vi "Markers.vi"(8 "error in (no error)":errorcluster, 10 "Subject Name":string, 11 ".NET Refnum in":refnum<k24>) -> (0 "error out":errorcluster, 2 "Markers Count":u32, 3 ".NET Reference out":refnum<k24>, 4 "Markers Name":string[](array[string]))   [LabVIEW 2024]
uses:
  C:/Users/ROAR/Documents/Rob Motor Assessment stuff/Labview/RobUST_3D_with_Unity_Control_PXI_Low_Level_Only_Streamlined/Vicon_files/ViconDataStreamSDK_DotNET.dll
  Vicon_files/ViconDataStreamSDK_DotNET.dll
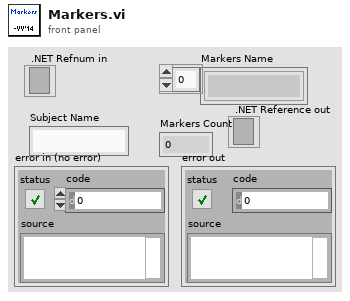
[diagram p1: front panel]
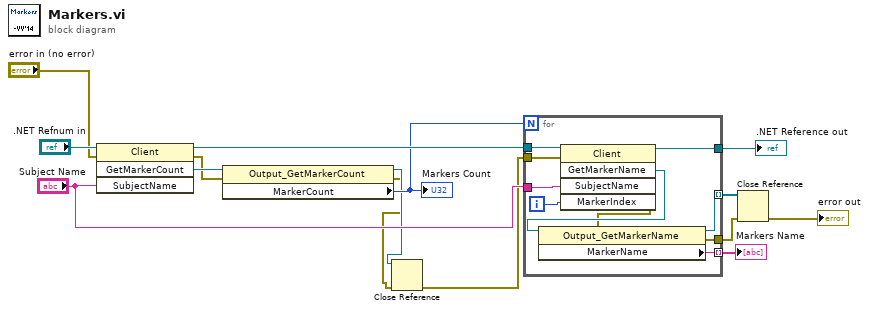
[diagram p0: block diagram]
diagram:
  n1 = invoke class="Client" method="GetMarkerCount"(reference=".NET Refnum in", error in="error in (no error)", "SubjectName"="Subject Name") -> (reference out=w14:refnum<k24>, error out=w7:errorcluster, "GetMarkerCount"=w10:refnum<k24>)  [unwired: 1 in, 1 out]
  n2 = property class="Output_GetMarkerCount"(reference=w10, error in=w7) -> (reference out=w6:refnum<k24>, error out=w5:errorcluster, "MarkerCount"=w11:u32)
  "Markers Count" <- w11
  n3 = Close Reference(reference=w6, error in (no error)=w5) -> (error out=w4:errorcluster)
  n4 = for {
    N: w11 -> [_]
    tunnel: w14 -> [w25]
    tunnel: "Subject Name" -> [w21]
    tunnel: [w22] -> w12 mode=indexing
    tunnel: [w20] -> w9
    tunnel: w4 -> [w19]
    tunnel: [w18] -> w3 mode=indexing
    tunnel: [w17] -> w2
    i -> [w24]
    n5 = invoke class="Client" method="GetMarkerName"(reference=w25, error in=w19, "SubjectName"=w21, "MarkerIndex"=w24) -> (reference out=w20:refnum<k24>, error out=w16:errorcluster, "GetMarkerName"=w23:refnum<k24>)  [unwired: 1 in, 2 out]
    n6 = property class="Output_GetMarkerName"(reference=w23, error in=w16) -> (reference out=w18:refnum<k24>, error out=w17:errorcluster, "MarkerName"=w22:string)
  }
  "Markers Name" <- w12
  ".NET Reference out" <- w9
  n7 = Close Reference(reference=w3, error in (no error)=w2) -> (error out=→"error out":errorcluster)
